vi "InitialTrayStatus.vi"(8 "error in (no error)":errorcluster, 11 "LaserDetect01 in":refnum<class "LaserDetect01.lvclass">) -> (0 "error out":errorcluster, 3 "LaserDetect01 out":refnum<class "LaserDetect01.lvclass">)   [LabVIEW 2019, in "LaserDetect01.lvclass"]
uses:
  LaserDetect01.lvclass
  FlowIOCtrl.lvclass
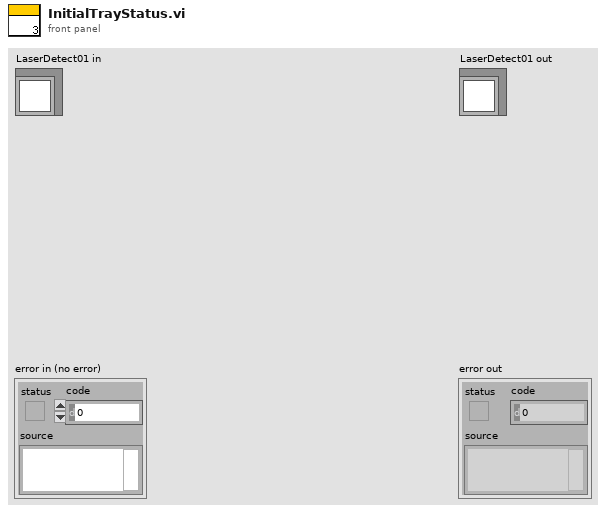
[diagram p1: front panel]
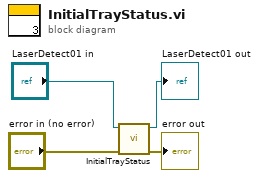
[diagram p0: block diagram]
diagram:
  n1 = call-parent "InitialTrayStatus.vi"("error in (no error)"="error in (no error)", "Station Action in"="LaserDetect01 in") -> ("error out"=→"error out":errorcluster, "Station Action out"=→"LaserDetect01 out":refnum<class "LaserDetect01.lvclass">)  [unwired: 8 in]
